vi "MainPC.vi"() -> ()   [LabVIEW 2017]
doc: "Use this template to build a simple state machine design pattern. Each state executes code and determines which state to transition to."
uses:
  Controls/UIState.ctl
  Controls/CommandsRT.ctl
panel:
  in  "Stop":bool
  in  "Pause":bool
  in  "Solution's moves":string
  in  "Start":bool
  in  "Exit":bool
  # "Rubik's Cube Solver"
  # "A myRIO hardware controls servos to turn an grip the cube.\n\nEnter a string of moves as \"U R U' D\" which solves a jumpled cube."
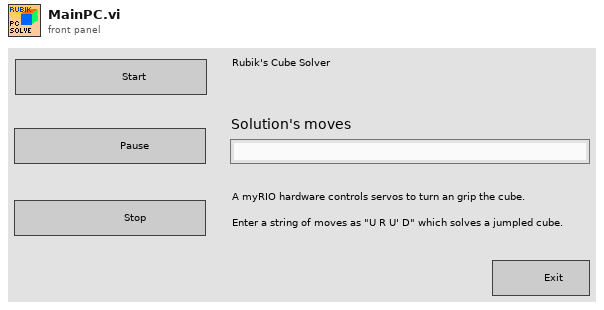
[diagram p1: front panel]
types:
  T1 = typedef "UIState.ctl" = enum16{"Wait for Event", "Initializing", "Starting", "Pausing", "Stopping", "Exiting"}
  T2 = typedef "CommandsRT.ctl" = enum16{"Initialize", "Start", "Pause", "Stop", "Exit"}
  T3 = typedef "DataStreamCluster.ctl" = cluster{"Commands":T2, variant}
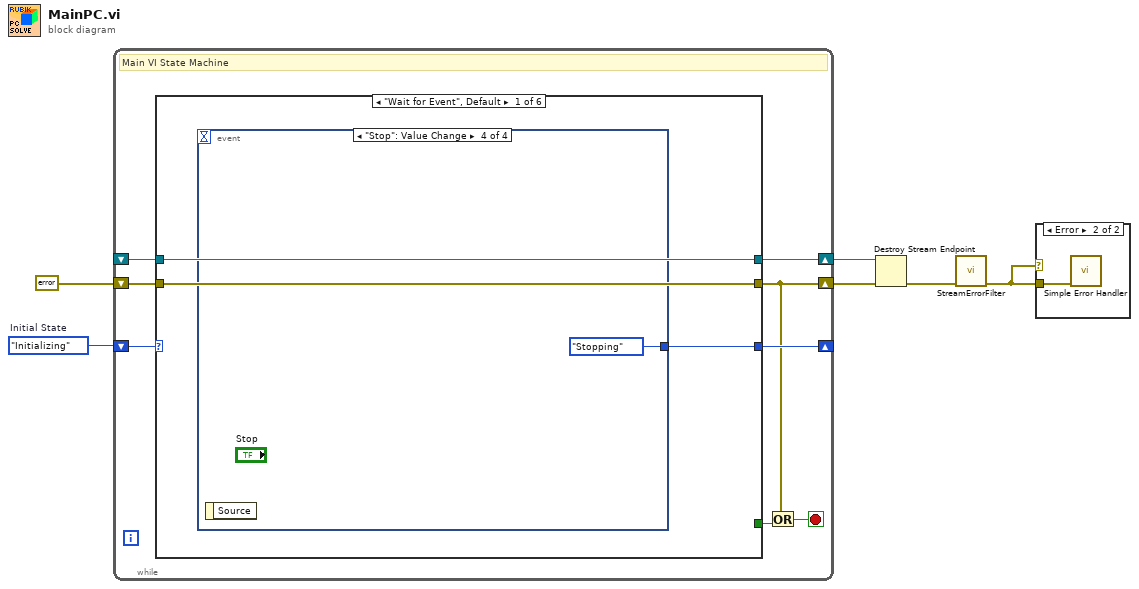
[diagram p0: block diagram]
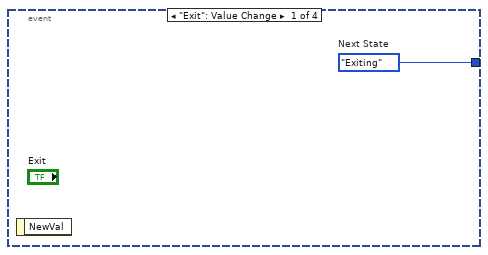
[diagram p3: hidden frame]
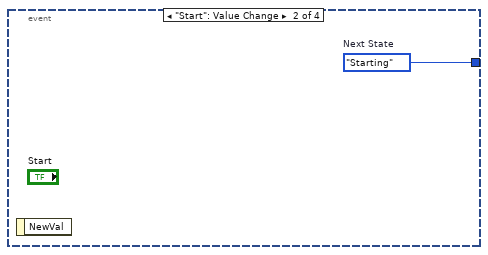
[diagram p4: hidden frame]
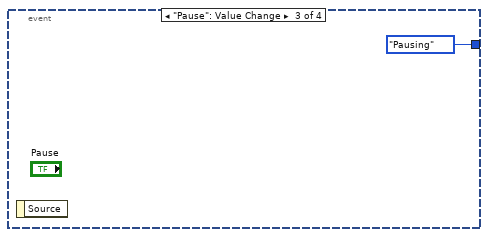
[diagram p5: hidden frame]
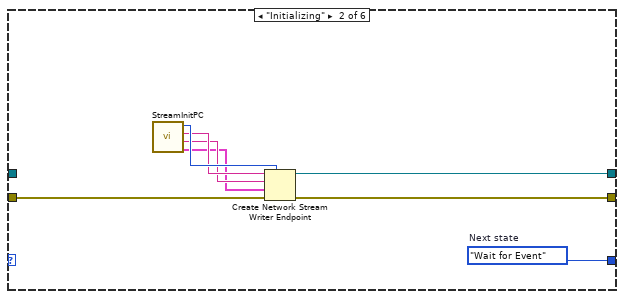
[diagram p6: hidden frame]
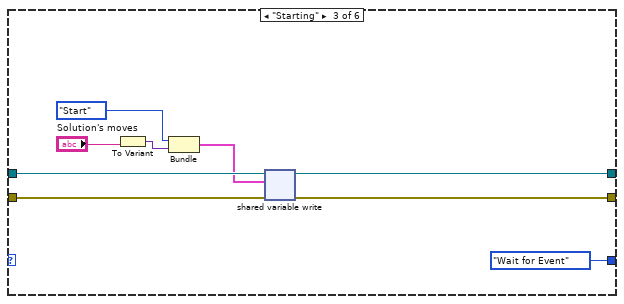
[diagram p7: hidden frame]
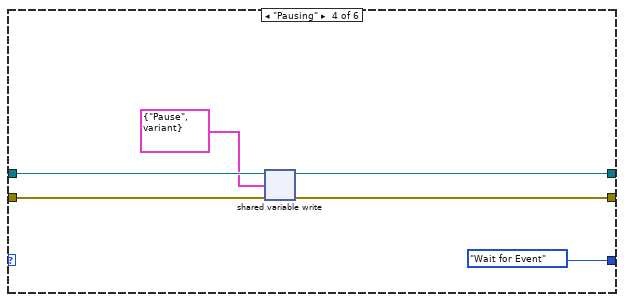
[diagram p8: hidden frame]
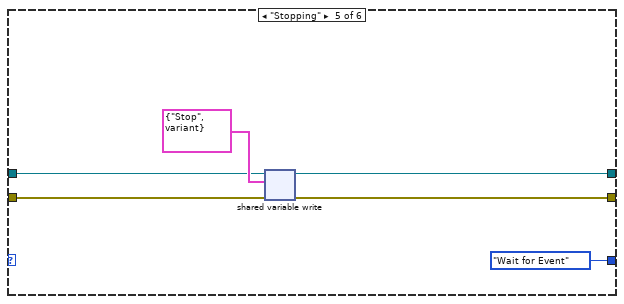
[diagram p9: hidden frame]
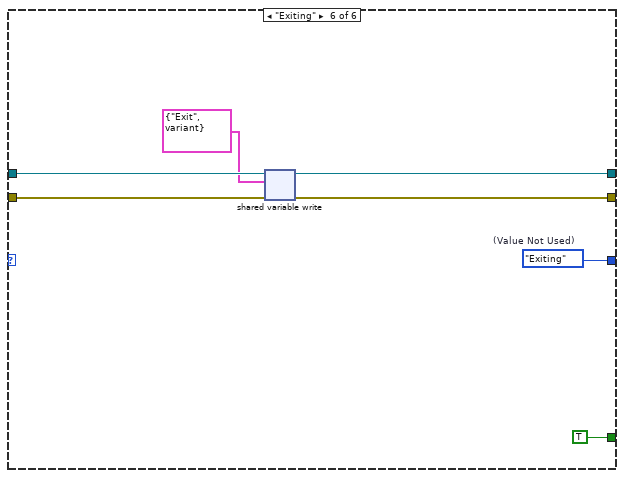
[diagram p10: hidden frame]
diagram:
  w6 = UIState."Initializing"  # Initial State
  n1 = while {
    shift-right: [w14] -> _
    shift-left: w6 -> [w11]
    shift-right: [w7] -> w4
    shift-left: errorcluster {"status"=FALSE, "code"=0, "source"=""} ("error constant") -> [w10]
    shift-right: [w9] -> w3
    shift-left: _ -> [w8]
    stop <- w12 stop-if-true
    # "Main VI State Machine"
    n2 = case shown="\"Wait for Event\", Default" w11 {
      tunnel: [w17 w29 UIState."Wait for Event" ("(Value Not Used)") UIState."Wait for Event" UIState."Wait for Event" ("(Value Not Used)") w57] -> w14
      tunnel: [_ _ _ _ _ TRUE ("Stop Loop?")] -> w13
      tunnel: [w15 w25 w36 w40 w49 w54] -> w7
      tunnel: w10 -> [w15 w23 w37 w41 w50 w55]
      tunnel: [w16 w24 w35 w42 w48 w53] -> w9
      tunnel: w8 -> [w16 _ w34 w43 w46 w52]
      frame "Wait for Event", Default {
        # "Wait for Event - Use an Event Structure to monitor the user interface for events that run different states of the state machine."
        n3 = event shown="[3] \"Stop\": Value Change" {
          selector: _ -> [_ _ _ _]
          dyn-events: _ -> [_ _ _ _]
          timeout: _ -> [_ _ _ _]
          tunnel: [w18 w19 UIState."Pausing" ("Next State") UIState."Stopping" ("Next State")] -> w17
          event "Exit": Value Change {
            w18 = UIState."Exiting"  # Next State
            n4 = event-data() -> ()  [unwired: 1 in, 1 out]
          }
          event "Start": Value Change {
            w19 = UIState."Starting"  # Next State
            n5 = event-data() -> ()  [unwired: 1 in, 1 out]
          }
          event "Pause": Value Change {
            n6 = event-data() -> ()  [unwired: 1 in, 1 out]
          }
          event "Stop": Value Change {
            n7 = event-data() -> ()  [unwired: 1 in, 1 out]
          }
        }
      }
      frame "Initializing" {
        w29 = UIState."Wait for Event"  # Next state
        # "Initialize - Initialize the application."
        n8 = call "StreamInitPC.vi"() -> ("data cluster"=w22:T3, "reader name"=w26:string, "writer name"=w27:string, "writer buffer size"=w28:i32)  [unwired: 4 in]
        n9 = Create Network Stream Writer Endpoint(7:w28, 8:w23, 9:w22, 10:w26, 11:w27) -> (0:w25:errorcluster, 3:w24:refnum<k21>)  [unwired: 2 in]
      }
      frame "Starting" {
        n10 = To Variant(anything="Solution's moves") -> (Variant=w31:variant)
        n11 = Bundle("Commands"=CommandsRT."Start", "Variant"=w31) -> (w30:cluster{"Commands":T2, "Variant":variant})  [unwired: 1 in]
        n12 = shared-variable-write(w34, w37, w30) -> (w35:refnum<k21>, w36:errorcluster)  [unwired: 1 in, 1 out]
      }
      frame "Pausing" {
        # "Exit - Exit the application."
        n13 = shared-variable-write(w43, w41, cluster{"Commands":T2, variant} {"Commands"=enum."Pause", variant} ("anything")) -> (w42:refnum<k21>, w40:errorcluster)  [unwired: 1 in, 1 out]
      }
      frame "Stopping" {
        n14 = shared-variable-write(w46, w50, cluster{"Commands":T2, variant} {"Commands"=enum."Stop", variant} ("anything")) -> (w48:refnum<k21>, w49:errorcluster)  [unwired: 1 in, 1 out]
      }
      frame "Exiting" {
        w57 = UIState."Exiting"  # (Value Not Used)
        n15 = shared-variable-write(w52, w55, cluster{"Commands":T2, variant} {"Commands"=enum."Exit", variant} ("anything")) -> (w53:refnum<k21>, w54:errorcluster)  [unwired: 1 in, 1 out]
      }
    }
    n16 = Or(x=w7, y=w13) -> (x .or. y?=w12:bool)
  }
  n17 = Destroy Stream Endpoint(8:w4, 11:w3) -> (0:w5:errorcluster)
  n18 = call "StreamErrorFilter.vi"("error in (no error)"=w5) -> ("error out"=w1:errorcluster)  [unwired: 10 in]
  n19 = case shown="Error" w1 {
    tunnel: w1 -> [_ w58]
    frame No Error {
    }
    frame Error {
      n20 = call <vilib>:"Simple Error Handler.vi"("error in (no error)"=w58) -> ()  [unwired: 4 in, 5 out]
    }
  }
